vi "Get Transactions.vi"(8 "error in (no error)":errorcluster, 11 "Statement in":refnum<class "Statement.lvclass">) -> (0 "error out":errorcluster, 2 "Transactions":refnum<class "Transaction.lvclass">[](array[class]), 3 "Statement out":refnum<class "Statement.lvclass">)   [LabVIEW 2018, in "Statement.lvclass"]
uses:
  Statement.lvclass
  Transaction/Transaction.lvclass
  Statement.lvclass/Statement.ctl
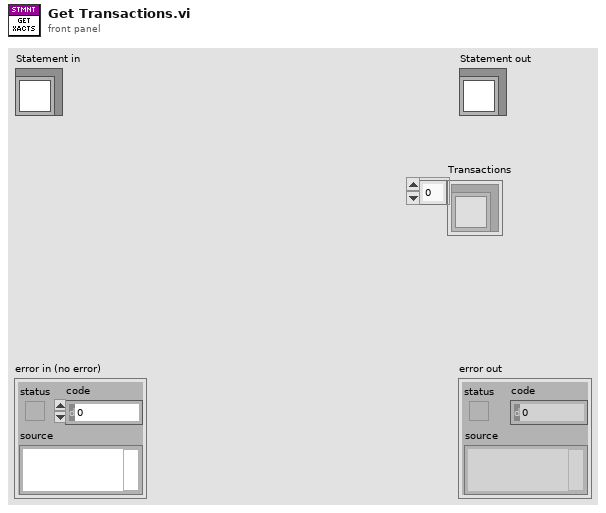
[diagram p1: front panel]
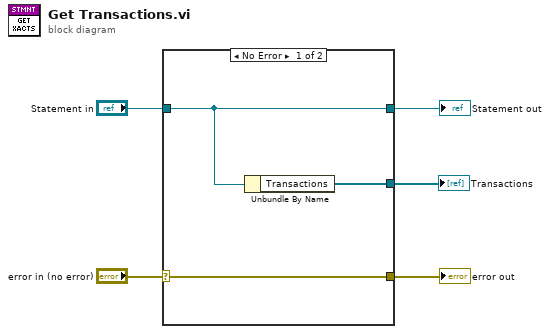
[diagram p0: block diagram]
diagram:
  n1 = case shown="No Error" "error in (no error)" {
    selector: "error in (no error)" -> [w8 w10]
    tunnel: [w8 w10] -> w4
    tunnel: [w7 w9] -> w2
    tunnel: "Statement in" -> [w7 w9]
    tunnel: [w6 _] -> w1
    frame No Error {
      n2 = Unbundle By Name(w7) -> ("Transactions"=w6:refnum<class "Transaction.lvclass">[])
    }
    frame Error {
    }
  }
  "error out" <- w4
  "Statement out" <- w2
  "Transactions" <- w1
